vi "Autonomous Independent.vi"() -> ()   [LabVIEW 2013]
doc: "This VI is called when autonomous begins, and will automatically be terminated when autonomous ends. You can carry out timed or sensor driven robot movement independently without needing to return to the caller."
uses:
  Robot Global Data.vi
  Events.vi
  <vilib>/Rock Robotics/WPI/Joystick/WPI_JoystickGetSetRefNum.vi
  <vilib>/Rock Robotics/WPI/RobotDrive/WPI_RobotDriveArcadeDrive_Standard(NoSaturation).vi
panel:
  out "Current Movement, for debugging":T1 {"Y Joystick Value" scale=1.0..-1.0; "X Joystick Value" scale=-1.0..1.0}
  in  "Array of robot movements":T2(array[cluster]) {"Y Joystick Value" scale=1.0..-1.0; "X Joystick Value" scale=-1.0..1.0}
  # "Be sure to right-click and choose Data Operations>>Make Current Value default if you want to save the array values with the VI"
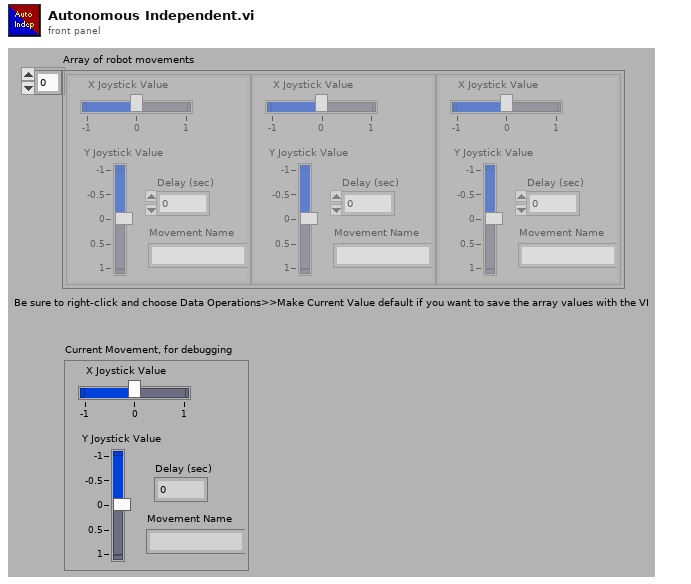
[diagram p1: front panel]
types:
  T1 = cluster{"X Joystick Value":dbl, "Y Joystick Value":dbl, "Delay (sec)":dbl, "Movement Name":string}
  T2 = cluster{"X Joystick Value":dbl, "Y Joystick Value":dbl, "Delay (sec)":dbl, "Movement Name":string}[]
  T3 = typedef "WPI_JoystickDevRef.ctl" = cluster{"Device":T4}
  T4 = typedef "WPI_JoystickDeviceEnum.ctl" = enum16{"USB 1", "USB 2", "USB 3", "USB 4", "Kinect 1", "Kinect 2"}
  T5 = cluster{"axis 1 (x)":dbl, "axis 2 (y)":dbl, "axis 3 (throttle)":dbl, "axis 4":dbl, "axis 5":dbl, "axis 6":dbl}
  T6 = cluster{"Drive Axis Translate":dbl, "Drive axis Forward Speed":dbl, "Drive axis Rotate":dbl, "Drive axis Tank right side":dbl, "axis 5":dbl, "axis 6":dbl}
  T7 = cluster{"Translate":dbl, "Forward Speed":dbl, "Rotate":dbl, "Tank right side":dbl, "axis 5":dbl, "axis 6":dbl}
  T8 = typedef "WPI_RobotDriveDevRef.ctl" = cluster{"DevStatus":errorcluster, "Motors[]":T9[], "Square Inputs":bool, "Max Output":dbl, "Isochronous":bool}
  T9 = typedef "WPI_MotorControlDeviceRef.ctl" = cluster{"DeviceStatus":errorcluster, "Type":enum16{"PWM", "CAN"}, "PWM":cluster{"Digital Module":T10, "PWM Channel":T11, "DeadBand":T12}, "CAN":cluster{"Device Number":u8, "Control Mode":T13, "Semaphore":T14, "Max Vout":dbl}, "Invert":bool, "TransformRef":T15, "InvTransformRef":T15}
  T10 = typedef "FPGA_TypedefDigitalModule.ctl" = enum16{"Digital Module 1", "Digital Module 2"}
  T11 = typedef "FPGA_DIOPWMChannel.ctl" = enum8{"PWM 1", "PWM 2", "PWM 3", "PWM 4", "PWM 5", "PWM 6", "PWM 7", "PWM 8", "PWM 9", "PWM 10", "Invalid"}
  T12 = typedef "WPI_PWMDeadband.ctl" = cluster{"Name":string, "maxPositivePwm":i32, "minPositivePwm":i32, "centerPwm":i32, "maxNegativePwm":i32, "minNegativePwm":i32, "angularRange":u16}
  T13 = typedef "WPI_CANJaguar_ControlMode.ctl" = enum8{"Percent VBus", "Current", "Speed", "Position", "Voltage"}
  T14 = typedef "Semaphore RefNum" = refnum<k1>
  T15 = typedef "WPI_PWMTransform_ConPane.ctl" = refnum<vi>
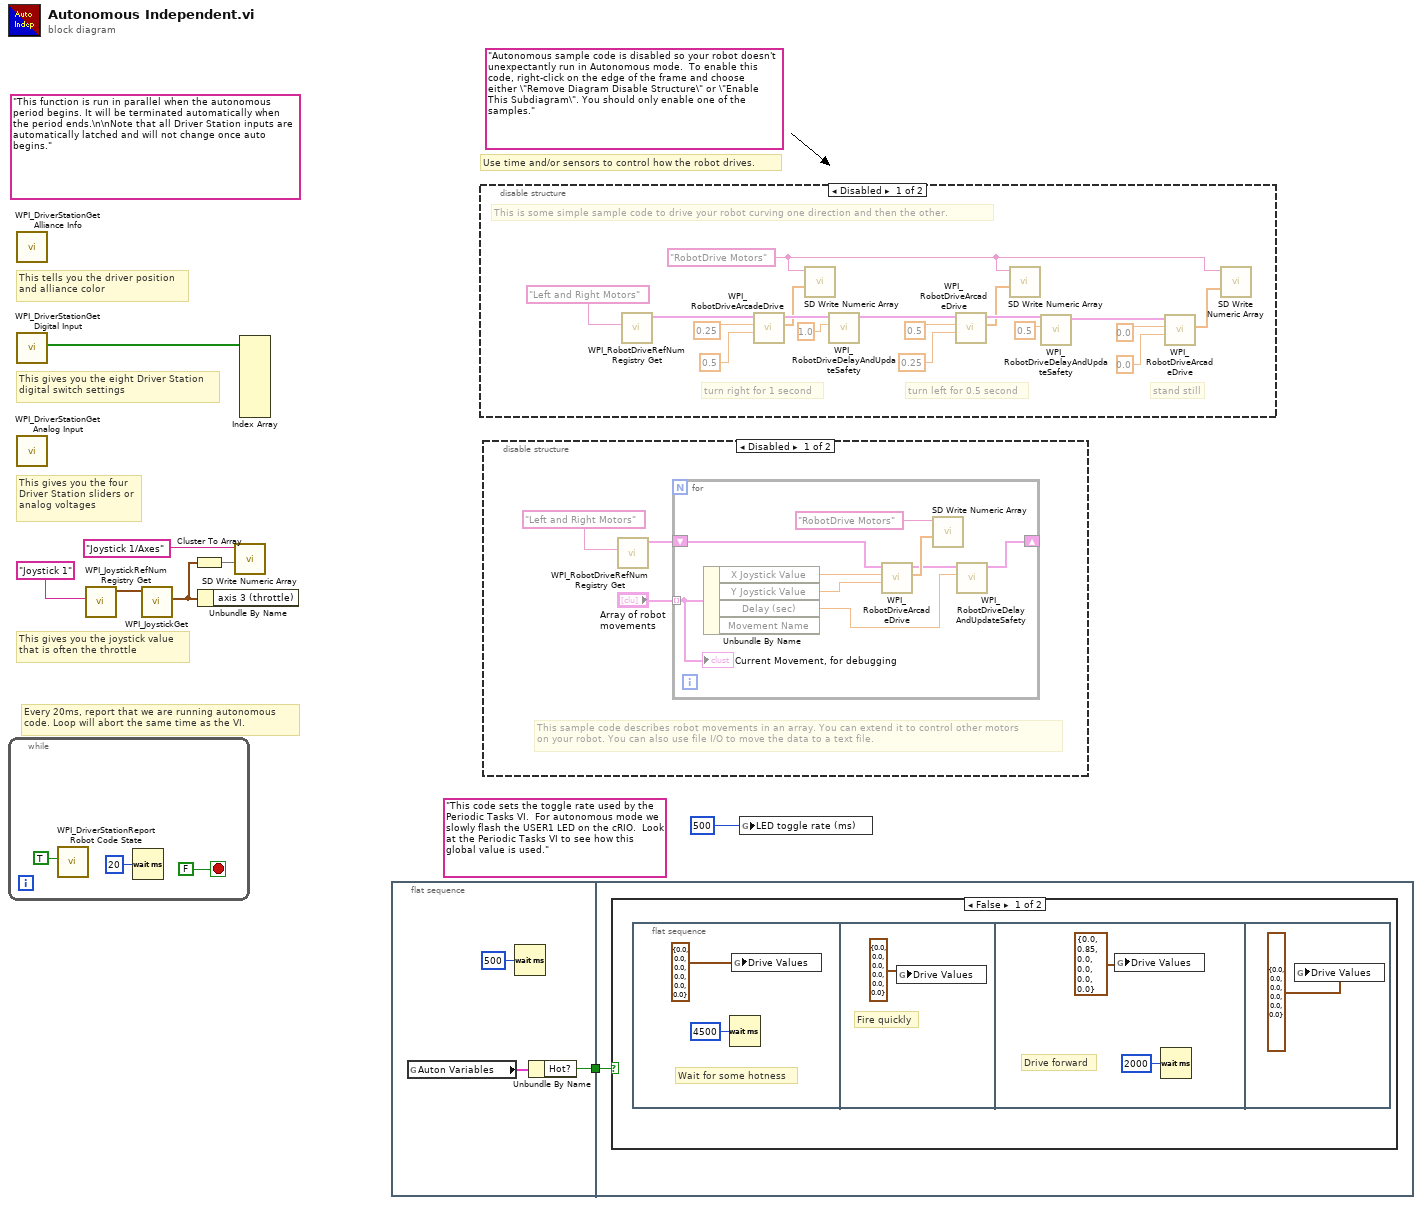
[diagram p0: block diagram]
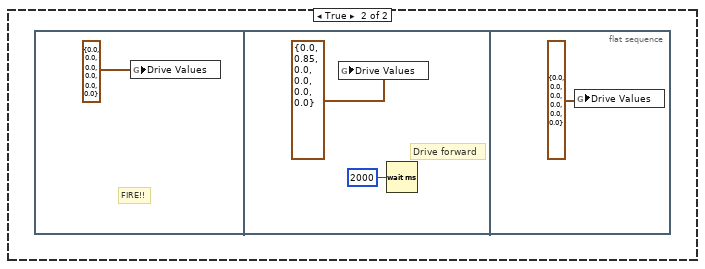
[diagram p2: hidden frame]
diagram:
  (unwired) "This code sets the toggle rate used by the Periodic Tasks VI.  For autonomous mode we slowly flash the USER1 LED on the cRIO.  Look at the Periodic Tasks VI to see how this global value is used."
  (unwired) "Autonomous sample code is disabled so your robot doesn't unexpectantly run in Autonomous mode.  To enable this code, right-click on the edge of the frame and choose either \"Remove Diagram Disable Structure\" or \"Enable This Subdiagram\". You should only enable one of the samples."
  (unwired) "This function is run in parallel when the autonomous period begins. It will be terminated automatically when the period ends.\n\nNote that all Driver Station inputs are automatically latched and will not change once auto begins."
  # "Every 20ms, report that we are running autonomous\ncode. Loop will abort the same time as the VI."
  # "This gives you the joystick value\nthat is often the throttle"
  # "Use time and/or sensors to control how the robot drives."
  # "This tells you the driver position\nand alliance color"
  # "This gives you the eight Driver Station\ndigital switch settings"
  # "This gives you the four\nDriver Station sliders or\nanalog voltages"
  n1 = while {
    stop <- FALSE stop-if-true
    n2 = call <vilib>:"WPI_DriverStationReport Robot Code State.vi"("Autonomous"=TRUE) -> ()  [unwired: 10 in, 1 out]
    n3 = Wait (ms)(milliseconds to wait=u32 20) -> ()  [unwired: 1 out]
  }
  n4 = call <vilib>:"WPI_DriverStationGet Alliance Info.vi"() -> ()  [unwired: 12 out]
  n5 = call <vilib>:"WPI_DriverStationGet Digital Input.vi"() -> ("Driver Station Digital Input (1-8)"=w8:bool[])  [unwired: 11 out]
  n6 = call <vilib>:"WPI_DriverStationGet Analog Input.vi"() -> ()  [unwired: 12 out]
  n7 = call <vilib>:"WPI_JoystickRefNum Registry Get.vi"("refnum name"="Joystick 1") -> ("JoystickDevRef"=w6:T3)  [unwired: 1 in, 9 out]
  n8 = call <vilib>:"WPI_JoystickGet.vi"("JoystickDevRef"=w6) -> ("Axes"=w3:T5)  [unwired: 1 in, 5 out]
  n9 = Cluster To Array(cluster=w3) -> (array=w4:dbl[])
  n10 = Unbundle By Name(w3) -> ()  [unwired: 1 out]
  n11 = call <vilib>:"SD Write Numeric Array.vi"("Numeric Array"=w4, "Name"="Joystick 1/Axes") -> ()  [unwired: 8 in, 2 out]
  n12 = Index Array(array=w8) -> ()  [unwired: 8 in, 8 out]
  n13 = flat-sequence {
    tunnel: [w13] -> w1
    tunnel: w1 -> [w15]
    frame #0 {
      n14 = global read "Events.vi" "Auton Variables"() -> (w14:cluster{"Hot?":bool})
      n15 = Wait (ms)(milliseconds to wait=u32 500) -> ()  [unwired: 1 out]
      n16 = Unbundle By Name(w14) -> ("Hot?"=w13:bool)
    }
    frame #1 {
      n17 = case shown="False" w15 {
        frame False {
          n18 = flat-sequence {
            frame #0 {
              # "Wait for some hotness"
              n19 = Wait (ms)(milliseconds to wait=u32 4500) -> ()  [unwired: 1 out]
              n20 = global write "Events.vi" "Drive Values"(T6 {"Drive Axis Translate"=0.0, "Drive axis Forward Speed"=0.0, "Drive axis Rotate"=0.0, "Drive axis Tank right side"=0.0, "axis 5"=0.0, "axis 6"=0.0} ("Drive Values")) -> ()
            }
            frame #1 {
              # "Fire quickly"
              n21 = global write "Events.vi" "Drive Values"(T6 {"Drive Axis Translate"=0.0, "Drive axis Forward Speed"=0.0, "Drive axis Rotate"=0.0, "Drive axis Tank right side"=0.0, "axis 5"=0.0, "axis 6"=0.0} ("Drive Values")) -> ()
            }
            frame #2 {
              # "Drive forward"
              n22 = global write "Events.vi" "Drive Values"(T6 {"Drive Axis Translate"=0.0, "Drive axis Forward Speed"=0.85, "Drive axis Rotate"=0.0, "Drive axis Tank right side"=0.0, "axis 5"=0.0, "axis 6"=0.0} ("Drive Values")) -> ()
              n23 = Wait (ms)(milliseconds to wait=u32 2000) -> ()  [unwired: 1 out]
            }
            frame #3 {
              n24 = global write "Events.vi" "Drive Values"(T7 {"Translate"=0.0, "Forward Speed"=0.0, "Rotate"=0.0, "Tank right side"=0.0, "axis 5"=0.0, "axis 6"=0.0} ("Drive Values")) -> ()
            }
          }
        }
        frame True {
          n25 = flat-sequence {
            frame #0 {
              # "FIRE!!"
              n26 = global write "Events.vi" "Drive Values"(T6 {"Drive Axis Translate"=0.0, "Drive axis Forward Speed"=0.0, "Drive axis Rotate"=0.0, "Drive axis Tank right side"=0.0, "axis 5"=0.0, "axis 6"=0.0} ("Drive Values")) -> ()
            }
            frame #1 {
              # "Drive forward"
              n27 = global write "Events.vi" "Drive Values"(T6 {"Drive Axis Translate"=0.0, "Drive axis Forward Speed"=0.85, "Drive axis Rotate"=0.0, "Drive axis Tank right side"=0.0, "axis 5"=0.0, "axis 6"=0.0} ("Drive Values")) -> ()
              n28 = Wait (ms)(milliseconds to wait=u32 2000) -> ()  [unwired: 1 out]
            }
            frame #2 {
              n29 = global write "Events.vi" "Drive Values"(T7 {"Translate"=0.0, "Forward Speed"=0.0, "Rotate"=0.0, "Tank right side"=0.0, "axis 5"=0.0, "axis 6"=0.0} ("Drive Values")) -> ()
            }
          }
        }
      }
    }
  }
  n30 = disable-structure shown="Disabled" {
    frame Disabled {
      w26 = "RobotDrive Motors" ("Name")
      # "This is some simple sample code to drive your robot curving one direction and then the other."
      # "stand still"
      # "turn left for 0.5 second"
      # "turn right for 1 second"
      n31 = call <vilib>:"WPI_RobotDriveRefNum Registry Get.vi"("refnum name"="Left and Right Motors") -> ("RobotDriveDevRef"=w30:T8)  [unwired: 1 in, 9 out]
      n32 = call-poly <vilib>:"WPI_RobotDriveArcadeDrive.vi"("Y axis value"=0.5 ("X axis value"), "X axis value"=0.25, "RobotDriveDevRef"=w30) -> ("Motor Values"=w29:dbl[], "RobotDriveDevRef"=w37:T8)  [unwired: 1 in, 6 out]
      n33 = call <vilib>:"SD Write Numeric Array.vi"("Numeric Array"=w29, "Name"=w26) -> ()  [unwired: 8 in, 2 out]
      n34 = call <vilib>:"WPI_RobotDriveDelayAndUpdateSafety.vi"("Delay (s)"=1.0, "RobotDriveDevRef"=w37) -> ("RobotDriveDevRef 2"=w36:T8)  [unwired: 8 in, 1 out]
      n35 = call-poly <vilib>:"WPI_RobotDriveArcadeDrive.vi"("Y axis value"=0.25 ("X axis value"), "X axis value"=0.5, "RobotDriveDevRef"=w36) -> ("Motor Values"=w28:dbl[], "RobotDriveDevRef"=w35:T8)  [unwired: 1 in, 6 out]
      n36 = call <vilib>:"SD Write Numeric Array.vi"("Numeric Array"=w28, "Name"=w26) -> ()  [unwired: 8 in, 2 out]
      n37 = call <vilib>:"WPI_RobotDriveDelayAndUpdateSafety.vi"("Delay (s)"=0.5, "RobotDriveDevRef"=w35) -> ("RobotDriveDevRef 2"=w34:T8)  [unwired: 8 in, 1 out]
      n38 = call-poly <vilib>:"WPI_RobotDriveArcadeDrive.vi"("Y axis value"=0.0 ("X axis value"), "X axis value"=0.0, "RobotDriveDevRef"=w34) -> ("Motor Values"=w27:dbl[])  [unwired: 1 in, 7 out]
      n39 = call <vilib>:"SD Write Numeric Array.vi"("Numeric Array"=w27, "Name"=w26) -> ()  [unwired: 8 in, 2 out]
    }
    frame Enabled {
    }
  }
  n40 = disable-structure shown="Disabled" {
    frame Disabled {
      # "This sample code describes robot movements in an array. You can extend it to control other motors\non your robot. You can also use file I/O to move the data to a text file."
      n41 = call <vilib>:"WPI_RobotDriveRefNum Registry Get.vi"("refnum name"="Left and Right Motors") -> ("RobotDriveDevRef"=w45:T8)  [unwired: 1 in, 9 out]
      n42 = for {
        shift-right: [w51] -> _
        shift-left: w45 -> [w52]
        tunnel: "Array of robot movements" -> [w47] mode=indexing
        n43 = Unbundle By Name(w47) -> ("X Joystick Value"=w50:dbl, "Y Joystick Value"=w49:dbl, "Delay (sec)"=w48:dbl)  [unwired: 1 out]
        n44 = call-poly <vilib>:"WPI_RobotDriveArcadeDrive.vi"("Y axis value"=w49, "X axis value"=w50, "RobotDriveDevRef"=w52) -> ("Motor Values"=w54:dbl[], "RobotDriveDevRef"=w53:T8)  [unwired: 1 in, 6 out]
        n45 = call <vilib>:"SD Write Numeric Array.vi"("Numeric Array"=w54, "Name"="RobotDrive Motors") -> ()  [unwired: 8 in, 2 out]
        n46 = call <vilib>:"WPI_RobotDriveDelayAndUpdateSafety.vi"("Delay (s)"=w48, "RobotDriveDevRef"=w53) -> ("RobotDriveDevRef 2"=w51:T8)  [unwired: 8 in, 1 out]
        "Current Movement, for debugging" <- w47
      }
    }
    frame Enabled {
    }
  }
  n47 = global write "Robot Global Data.vi" "LED toggle rate (ms)"(u32 500 ("LED ms toggle rate")) -> ()
